vi "Quadrant photodiode read.vi"(6 "Sensor Number\n(ignored)":dbl, 8 "number of readings\n to average":i32=1, 9 "Mode":enum16{"Start", "Read", "End"}(ring)) -> (0 "error out":errorcluster, 1 "Y position":dbl, 2 "X position":dbl, 3 "Power":dbl)   [LabVIEW 2015]
doc: "Operates the ThorLabs PDQ80S1 quandrant photodiode detector. Call with Mode=Start to initiate scanning; Mode=Read to read the detector; Mode=End to stop. Requires the home-made PDQ80S1.dll be located in the same directory as the VI."
uses:
  <vilib>/DAQmx/read.llb/DAQmx Read (Analog 2D DBL NChan NSamp).vi
  <vilib>/Analysis/baseanly.llb/Mean (DBL).vi
  h-nu-ixon/QPD config globals.vi
  <vilib>/DAQmx/create/channels.llb/DAQmx Create Channel (AI-Voltage-Basic).vi
  <vilib>/DAQmx/configure/timing.llb/DAQmx Timing (Sample Clock).vi
  <vilib>/DAQmx/miscellaneous.llb/DAQmx Fill In Error Info.vi
  <vilib>/Analysis/NI_AALBase.lvlib
panel:
  out "Sampling rate (s-1)":dbl=100.0 format="%0.2f"
  out "A-to-D channels\nfor x, y, power, supply":tag="Dev2/ai0:3"
  out "Supply voltage":dbl
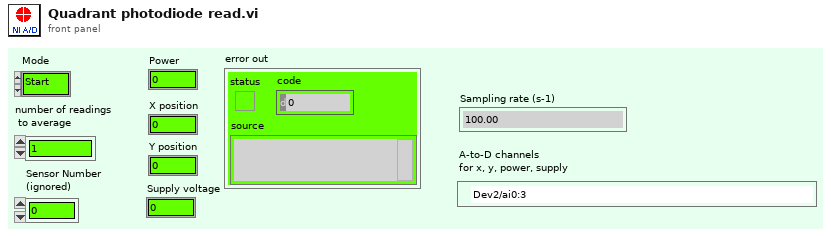
[diagram p1: front panel]
types:
  T1 = cluster{"[0]":dbl, "[1]":dbl, "[2]":dbl, "[3]":dbl, "[4]":dbl, "[5]":dbl, "[6]":dbl, "[7]":dbl, "[8]":dbl}
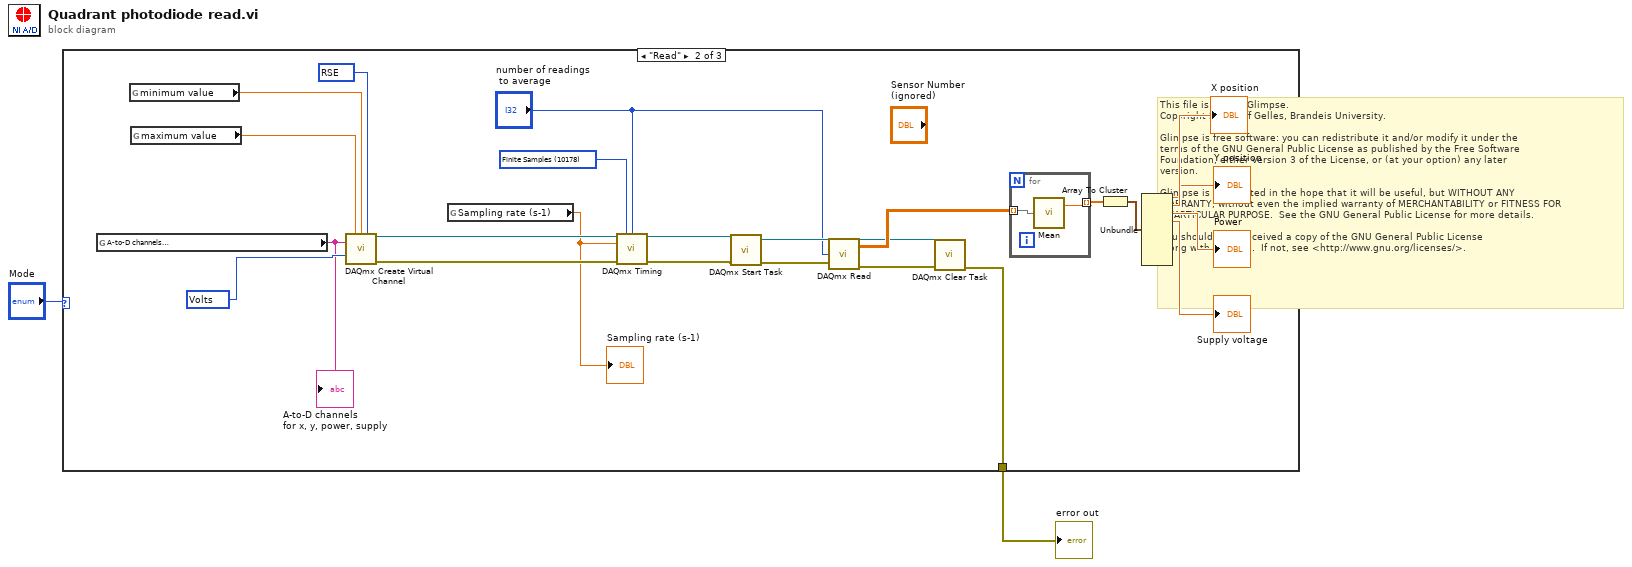
[diagram p0: block diagram]
diagram:
  # "This file is part of Glimpse. \nCopyright 2014 Jeff Gelles, Brandeis University.    \n\nGlimpse is free software: you can redistribute it and/or modify it under the \nterms of the GNU General Public License as published by the Free Software \nFoundation, either version 3 of the License, or (at your option) any later \nversion.\n\nGlimpse is distributed in the hope that it will be useful, but WITHOUT ANY \nWARRANTY; without even the implied warranty of MERCHANTABILITY or FITNESS FOR \nA PARTICULAR PURPOSE.  See the GNU General Public License for more details.\n\nYou should have received a copy of the GNU General Public License\nalong with Glimpse.  If not, see <http://www.gnu.org/licenses/>."
  n1 = case shown="\"Read\"" "Mode" {
    tunnel: [_ w17 _] -> w1
    frame "Start", Default {
    }
    frame "Read" {
      w13 = 10083 items=["default"=-1, "RSE"=10083, "NRSE"=10078, "Differential"=10106, "Pseudodifferential"=12529] ("input terminal configuration")
      w14 = 10178 items=["Finite Samples"=10178, "Continuous Samples"=10123, "Hardware Timed Single Point"=12522] ("sample mode")
      w16 = 10348 items=["Volts"=10348, "From Custom Scale"=10065] ("units")
      n2 = global read "QPD config globals.vi" "A-to-D channels\nfor x, y, power, supply"() -> (w7:tag)
      "A-to-D channels\nfor x, y, power, supply" <- w7
      n3 = global read "QPD config globals.vi" "minimum value"() -> (w5:dbl)
      n4 = global read "QPD config globals.vi" "maximum value"() -> (w6:dbl)
      n5 = call-poly <vilib>:"DAQmx Create Virtual Channel.vi"("maximum value"=w6, "minimum value"=w5, "input terminal configuration"=w13, "physical channels"=w7, "units"=w16) -> ("task out"=w15:refnum<k21>, "error out"=w12:errorcluster)  [unwired: 4 in, 5 out]
      n6 = global read "QPD config globals.vi" "Sampling rate (s-1)"() -> (w4:dbl)
      "Sampling rate (s-1)" <- w4
      n7 = call-poly <vilib>:"DAQmx Timing.vi"("task/channels in"=w15, "sample mode"=w14, "samples per channel"="number of readings\n to average", "rate"=w4) -> ("task out"=w11:refnum<k21>)  [unwired: 3 in, 8 out]
      n8 = call <vilib>:"DAQmx Start Task.vi"("task/channels in"=w11, "error in"=w12) -> ("task out"=w20:refnum<k21>, "error out"=w21:errorcluster)  [unwired: 12 out]
      n9 = call-poly <vilib>:"DAQmx Read.vi"("task/channels in"=w20, "number of samples per channel"="number of readings\n to average", "error in"=w21) -> ("task out"=w18:refnum<k21>, "data"=w25:dbl[][], "error out"=w19:errorcluster)  [unwired: 1 in, 9 out]
      n10 = call <vilib>:"DAQmx Clear Task.vi"("task in"=w18, "error in"=w19) -> ("error out"=w17:errorcluster)  [unwired: 13 out]
      n11 = for {
        tunnel: w25 -> [w27] mode=indexing
        tunnel: [w26] -> w24 mode=indexing
        n12 = call-poly <vilib>:"Mean.vi"("X"=w27) -> ("mean"=w26:dbl)  [unwired: 1 out]
      }
      n13 = Array To Cluster(array=w24) -> (cluster=w23:T1)
      n14 = Unbundle(w23) -> ("[0]"=→"Y position":dbl, "[1]"=→"X position":dbl, "[2]"=→"Power":dbl, "[3]"=→"Supply voltage":dbl)  [unwired: 5 out]
    }
    frame "End" {
    }
  }
  "error out" <- w1
